vi "Enqueue User Que (Array).vi"(6 "モード(Normal)":enum16{"Normal", "Lossy", "OppositeEnd"}(ring), 7 "コマンド[]":string[](array[string]), 8 "エラー入力（エラーなし）":errorcluster, 9 "タイムアウト（ms）（-1）":i32=-1, 10 "バリアント[]":variant[](array[variant]), 11 "queVariant":refnum<queue>) -> (0 "エラー出力":errorcluster, 1 "timeout/overflow?":bool, 3 "queVariant(copy)":refnum<queue>)   [LabVIEW 2014]
uses:
  QueData.ctl
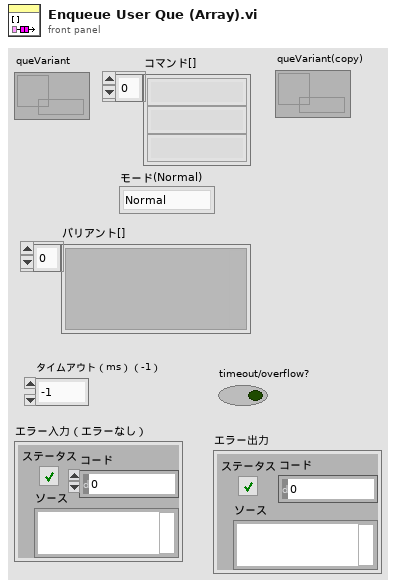
[diagram p1: front panel]
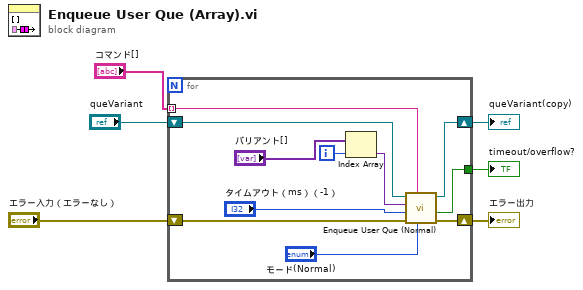
[diagram p0: block diagram]
diagram:
  n1 = for {
    tunnel: [w8] -> w6
    shift-right: [w7] -> w4
    shift-left: "queVariant" -> [w14]
    shift-right: [w11] -> w2
    shift-left: "エラー入力（エラーなし）" -> [w12]
    tunnel: "コマンド[]" -> [w17] mode=indexing
    i -> [w15]
    n2 = Index Array(array="バリアント[]", index=w15) -> (element=w13:variant)
    n3 = call "Enqueue User Que (Normal).vi"("モード(Normal)"="モード(Normal)", "コマンド"=w17, "エラー入力（エラーなし）"=w12, "タイムアウト（ms）（-1）"="タイムアウト（ms）（-1）", "バリアント"=w13, "queVariant"=w14) -> ("エラー出力"=w11:errorcluster, "timeout/overflow?"=w8:bool, "queVariant(copy)"=w7:refnum<queue>)  [unwired: 3 in]
  }
  "timeout/overflow?" <- w6
  "エラー出力" <- w2
  "queVariant(copy)" <- w4
